vi "AllowContinuousPressureAcquisition.vi"() -> ()   [LabVIEW 2012]
panel:
  in  "AllowContinuousPressureAcqusition":bool
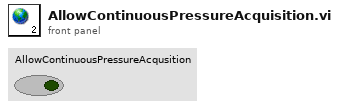
[diagram p1: front panel]
diagram:
